vi "SN_Check.vi"(8 "error in":errorcluster, 9 "PSU":string, 10 "OPID":string, 11 "SN":string) -> (0 "error out":errorcluster, 3 "pass?":bool)   [LabVIEW 2013]
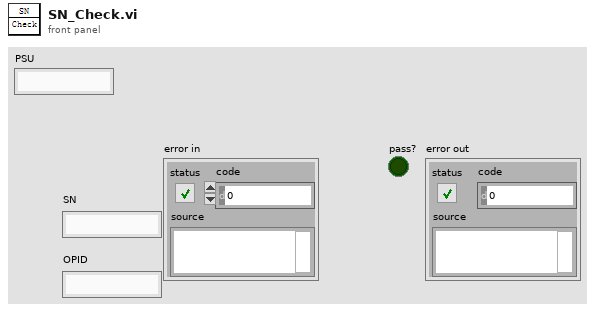
[diagram p1: front panel]
types:
  T1 = enum16{"open", "replace", "create", "open or create", "replace or create", "replace or create with confirmation"}
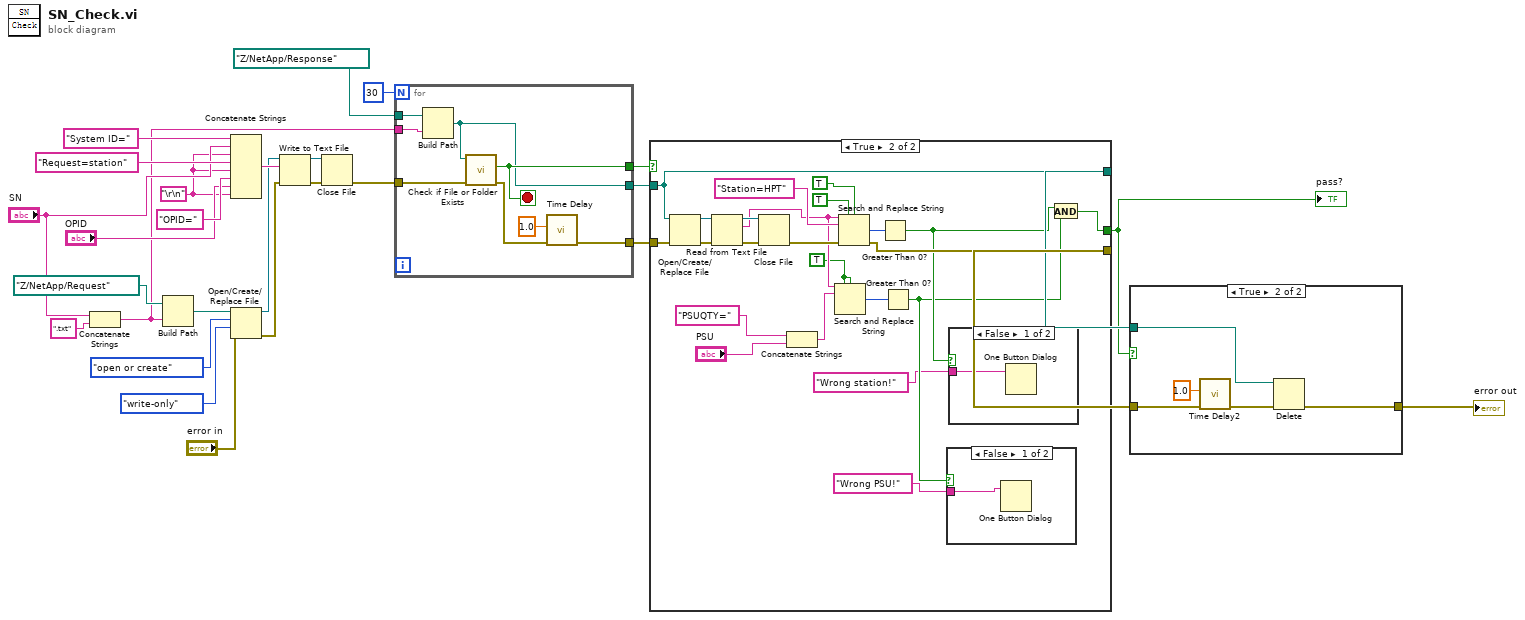
[diagram p0: block diagram]
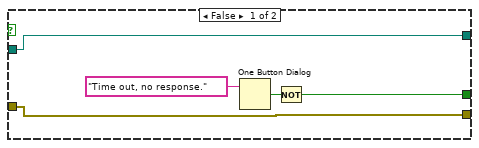
[diagram p3: hidden frame]
diagram:
  w2 = "\r\n"
  n1 = Concatenate Strings("SN", ".txt" ("string")) -> (w11:string)
  n2 = Build Path(base path=path "Z:/NetApp/Request", name or relative path=w11) -> (appended path=w20:path)
  n3 = Concatenate Strings("System ID=" ("string"), "SN", w2, "Request=station" ("string"), w2, "OPID=" ("string"), "OPID", w2) -> (w19:string)
  n4 = Open/Create/Replace File(file path (use dialog)=w20, error in="error in", operation (0:open)=T1."open or create", access (0:read/write)=enum16{"read/write", "read-only", "write-only"}."write-only") -> (refnum out=w18:refnum<file>, error out=w17:errorcluster)  [unwired: 2 in, 1 out]
  n5 = Write to Text File(file (use dialog)=w18, text=w19, error in=w17) -> (refnum out=w24:refnum<file>, error out=w23:errorcluster)  [unwired: 1 in, 1 out]
  n6 = Close File(refnum=w24, error in=w23) -> (error out=w13:errorcluster)  [unwired: 1 out]
  n7 = for {
    N: 30 -> [_]
    tunnel: w13 -> [w36]
    tunnel: path "Z:/NetApp/Response" ("base path") -> [w35]
    tunnel: w11 -> [w34]
    tunnel: [w31] -> w9
    tunnel: [w30] -> w8
    tunnel: [w29] -> w7
    stop <- w31 stop-if-true
    n8 = Build Path(base path=w35, name or relative path=w34) -> (appended path=w30:path)
    n9 = call <vilib>:"Check if File or Folder Exists.vi"("error in (no error)"=w36, "path"=w30) -> ("error out"=w32:errorcluster, "file or folder exists?"=w31:bool)  [unwired: 7 in, 1 out]
    n10 = call "Time Delay"("error in (no error)"=w32, "Delay Time (s)"=1.0) -> ("error out"=w29:errorcluster)  [unwired: 9 in]
  }
  n11 = case shown="True" w9 {
    tunnel: [w39 w46] -> w1
    tunnel: w8 -> [w37 w53]
    tunnel: w7 -> [w38 w60]
    tunnel: [w38 w54] -> w5
    tunnel: [w37 w53] -> w4
    frame False {
      n12 = One Button Dialog(message="Time out, no response.") -> (true=w40:bool)  [unwired: 1 in]
      n13 = Not(x=w40) -> (.not. x?=w39:bool)
    }
    frame True {
      w51 = TRUE ("replace all? (F)")
      n14 = Open/Create/Replace File(file path (use dialog)=w53, error in=w60) -> (refnum out=w62:refnum<file>, error out=w61:errorcluster)  [unwired: 4 in, 1 out]
      n15 = Read from Text File(file (use dialog)=w62, error in=w61) -> (refnum out=w64:refnum<file>, text=w52:string, error out=w63:errorcluster)  [unwired: 2 in, 1 out]
      n16 = Close File(refnum=w64, error in=w63) -> (error out=w56:errorcluster)  [unwired: 1 out]
      n17 = Concatenate Strings("PSUQTY=" ("search string"), "PSU") -> (w48:string)
      n18 = Search and Replace String(replace all?=w51, case sensitive?=w51, input string=w52, search string=w48) -> (number of replacements=w50:i32)  [unwired: 4 in, 3 out]
      n19 = Search and Replace String(replace all?=TRUE ("replace all? (F)"), case sensitive?=TRUE ("ignore case? (F)"), input string=w52, search string="Station=HPT", error in=w56) -> (number of replacements=w55:i32, error out=w54:errorcluster)  [unwired: 3 in, 2 out]
      n20 = Greater Than 0?(x=w55) -> (x > 0?=w45:bool)
      n21 = Greater Than 0?(x=w50) -> (x > 0?=w44:bool)
      n22 = case shown="False" w44 {
        tunnel: "Wrong PSU!" ("message") -> [w65 _]
        frame False {
          n23 = One Button Dialog(message=w65) -> ()  [unwired: 1 in, 1 out]
        }
        frame True {
        }
      }
      n24 = case shown="False" w45 {
        tunnel: "Wrong station!" ("message") -> [w66 _]
        frame False {
          n25 = One Button Dialog(message=w66) -> ()  [unwired: 1 in, 1 out]
        }
        frame True {
        }
      }
      n26 = And(x=w45, y=w44) -> (x .and. y?=w46:bool)
    }
  }
  "pass?" <- w1
  n27 = case shown="True" w1 {
    tunnel: w5 -> [w67 w72]
    tunnel: w4 -> [_ w71]
    tunnel: [w67 w70] -> w3
    frame False {
    }
    frame True {
      n28 = call "Time Delay2"("error in (no error)"=w72, "Delay Time (s)"=1.0) -> ("error out"=w68:errorcluster)  [unwired: 9 in]
      n29 = Delete(path (use dialog)=w71, error in=w68) -> (error out=w70:errorcluster)  [unwired: 3 in, 2 out]
    }
  }
  "error out" <- w3
